vi "Status Faults.vi"(0 "VISA resource name":refnum<visa-resource-name>, 1 "Fast Comms (F)":bool, 2 "Retry Attempts (0)":i32 min=0, 11 "error in (no error)":errorcluster) -> (4 "VISA resource name out":refnum<visa-resource-name>, 6 "Upper Pressure Fault":bool, 8 "Lower Pressure Fault":bool, 10 "Motor Stall Fault":bool, 15 "error out":errorcluster)   [LabVIEW 2020, in "driver_chromtech_nextgen_pump.lvlib"]
doc: "Query the instrument for any current faults."
uses:
  driver_chromtech_nextgen_pump.lvlib
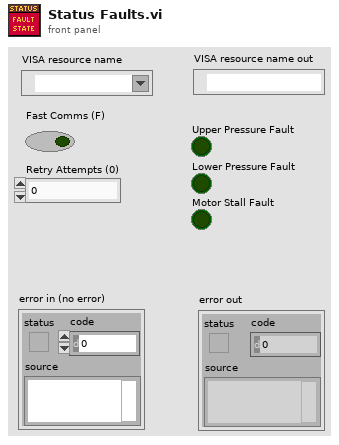
[diagram p1: front panel]
types:
  T1 = cluster{"Flow rate":dbl, "Running":bool, "Pressure Comp":i32, "Head ID":string, "Upper Pressure Fault":bool, "Lower Pressure Fault":bool, "In Prime":bool, "Keypad Enabled":bool, "Motor Stall Fault":bool}
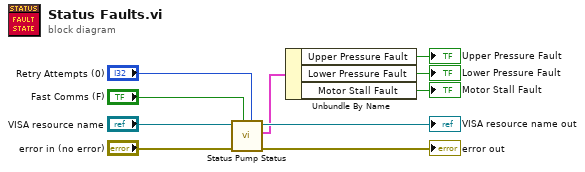
[diagram p0: block diagram]
diagram:
  n1 = call "Status Pump Status.vi"("Retry Attempts (0)"="Retry Attempts (0)", "Fast Comms (F)"="Fast Comms (F)", "error in (no error)"="error in (no error)", "VISA resource name"="VISA resource name") -> ("error out"=→"error out":errorcluster, "Status Cluster"=w5:T1, "VISA resource name out"=→"VISA resource name out":refnum<visa-resource-name>)  [unwired: 5 in]
  n2 = Unbundle By Name(w5) -> ("Upper Pressure Fault"=→"Upper Pressure Fault":bool, "Lower Pressure Fault"=→"Lower Pressure Fault":bool, "Motor Stall Fault"=→"Motor Stall Fault":bool)
